vi "写入硬件COM口.vi"(8 "error in (no error)":errorcluster caption="错误输入（无错误）", 10 "硬件COM口":refnum<visa-resource-name>, 11 "硬件输入":refnum<class "硬件.lvclass">) -> (0 "error out":errorcluster caption="错误输出", 3 "硬件输出":refnum<class "硬件.lvclass">)   [LabVIEW 2015, in "硬件.lvlib" / "硬件.lvclass"]
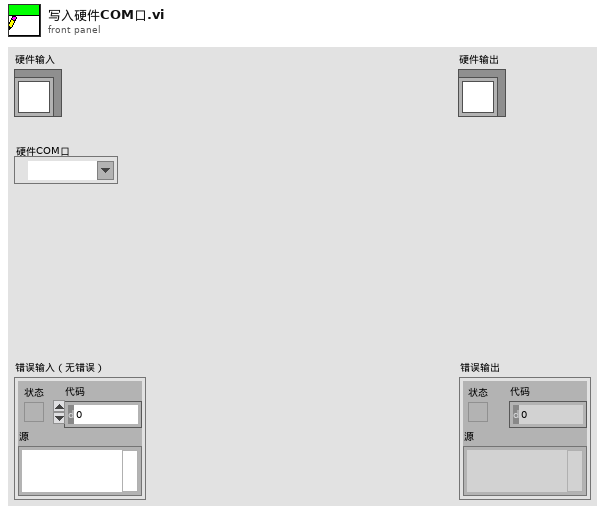
[diagram p1: front panel]
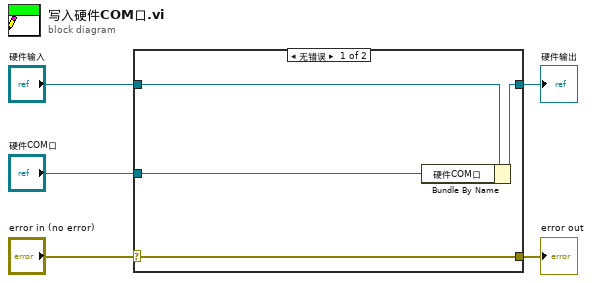
[diagram p0: block diagram]
diagram:
  n1 = case shown="无错误" "error in (no error)" {
    selector: "error in (no error)" -> [w9 w10]
    tunnel: [w9 w10] -> w4
    tunnel: [w7 w11] -> w2
    tunnel: "硬件输入" -> [w8 w11]
    tunnel: "硬件COM口" -> [w6 _]
    frame No Error {
      n2 = Bundle By Name(cluster=w8, "硬件COM口"=w6) -> (w7:refnum<class "硬件.lvclass">)
    }
    frame Error {
    }
  }
  "error out" <- w4
  "硬件输出" <- w2
